vi "Init SEQ from Builder.vi"(8 "error in":errorcluster, 11 "SEQ in":refnum<class "SEQ.lvclass">) -> (0 "error out":errorcluster, 3 "SEQ out":refnum<class "SEQ.lvclass">)   [LabVIEW 2012, in "Sequence Composition.lvlib" / "SEQ.lvclass"]
doc: "Initialize a sequence using the builder class."
uses:
  SEQ.lvclass
  Sequence Factory/Sequence Builder.lvclass
panel:
  in  "Builder":refnum<class "Sequence Builder.lvclass">
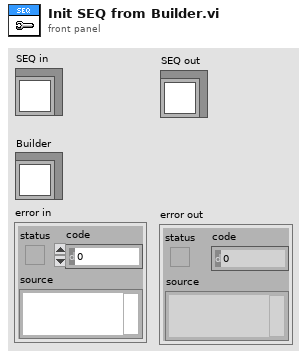
[diagram p1: front panel]
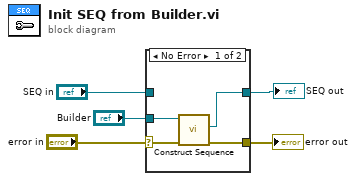
[diagram p0: block diagram]
diagram:
  n1 = case shown="No Error" "error in" {
    selector: "error in" -> [w7 w11]
    tunnel: [w6 w11] -> w4
    tunnel: [w8 w10] -> w2
    tunnel: "SEQ in" -> [_ w10]
    tunnel: "Builder" -> [w9 _]
    frame No Error {
      n2 = call-dynamic "Construct Sequence.vi"("error in"=w7, "Sequence Builder in"=w9) -> ("error out"=w6:errorcluster, "New Sequence"=w8:refnum<class "SEQ.lvclass">)  [unwired: 7 in, 1 out]
    }
    frame Error {
    }
  }
  "error out" <- w4
  "SEQ out" <- w2
